vi "Create.vi"(8 "error in (no error)":errorcluster, 10 "SPI #":T1=-1) -> (0 "error out":errorcluster, 3 "SPI out":refnum<class "SPI.lvclass">)   [LabVIEW 2020, in "CTI.lvlib" / "SPI.lvclass"]
uses:
  SPI.lvclass
  SPI Number.ctl
  SPI.lvclass/SPI.ctl
  CTI.lvlib
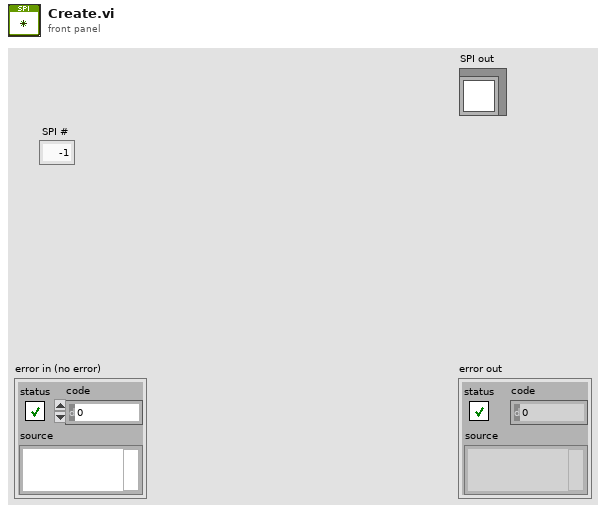
[diagram p1: front panel]
types:
  T1 = typedef "CTI.lvlib/SPI Number.ctl" = i8
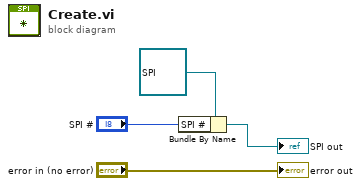
[diagram p0: block diagram]
diagram:
  n1 = Bundle By Name(cluster=refnum<class "SPI.lvclass"> refnum ("SPI in"), "SPI #"="SPI #") -> (→"SPI out":refnum<class "SPI.lvclass">)
  "error out" <- "error in (no error)"
